vi "Shutdown.vi"(8 "error in":errorcluster, 11 "TCP master in":refnum<class "SMSD Master.lvclass">) -> (0 "error out":errorcluster)   [LabVIEW 2021, in "SMSD Master.lvclass"]
doc: "Closes the TCP connection stored in the class."
uses:
  SMSD Master.lvclass
  SMSD Master.lvclass/SMSD Master.ctl
  Transmission Data Unit/SMSD/SMSD ADU.lvclass/SMSD ADU.ctl
  Transmission Data Unit/SMSD/SMSD ADU.lvclass
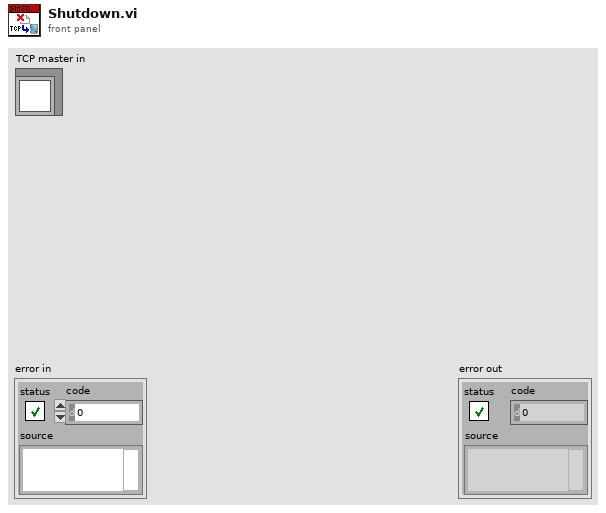
[diagram p1: front panel]
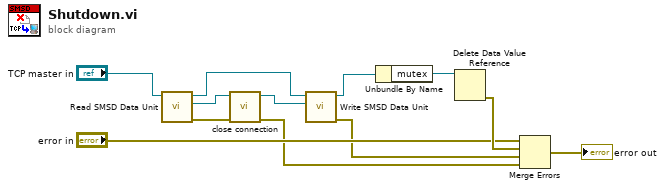
[diagram p0: block diagram]
diagram:
  n1 = call "Read SMSD Data Unit.vi"("SMSD Master in"="TCP master in") -> ("error out"=w10:errorcluster, "IP Data Unit"=w9:refnum<class "SMSD ADU.lvclass">, "SMSD Master out"=w11:refnum<class "SMSD Master.lvclass">)  [unwired: 8 in]
  n2 = call "close connection.vi"("error in"=w10, "TCP master in"=w9) -> ("error out"=w2:errorcluster, "TCP master out"=w8:refnum<class "SMSD ADU.lvclass">)  [unwired: 8 in]
  n3 = call "Write SMSD Data Unit.vi"("IP Data Unit"=w8, "SMSD Master in"=w11) -> ("error out"=w3:errorcluster, "SMSD Master out"=w4:refnum<class "SMSD Master.lvclass">)  [unwired: 8 in]
  n4 = Unbundle By Name(w4) -> ("mutex"=w7:refnum<data-value>)
  n5 = Delete Data Value Reference(data value reference=w7) -> (error out=w6:errorcluster)  [unwired: 1 in, 1 out]
  n6 = Merge Errors("error in", w6, w3, w2) -> (→"error out":errorcluster)
